vi "Accel math.vi"(4 "Numeric":i32, 8 "Base Accels 2":dbl[][](array[numeric]), 11 "Six Plane Accels 2":dbl[][](array[numeric])) -> (3 "Final Accel Values":dbl[][](array[numeric]))   [LabVIEW 2013]
uses:
  <vilib>/Analysis/NI_AALBase.lvlib
  <vilib>/Analysis/baseanly.llb/Real A x B.vi
  <vilib>/Analysis/baseanly.llb/Real Inverse Matrix.vi
panel:
  out "Final Accel Values 1":dbl[][](array[numeric])
  out "Numeric 4":dbl
  out "Numeric 2":dbl
  out "Numeric 3":dbl
  out "Final Accel Values 5":dbl[][](array[numeric])
  out "Final Accel Values 4":dbl[][](array[numeric])
  out "Final Accel Values 3":dbl[][](array[numeric])
  out "Final Accel Values 2":dbl[][](array[numeric])
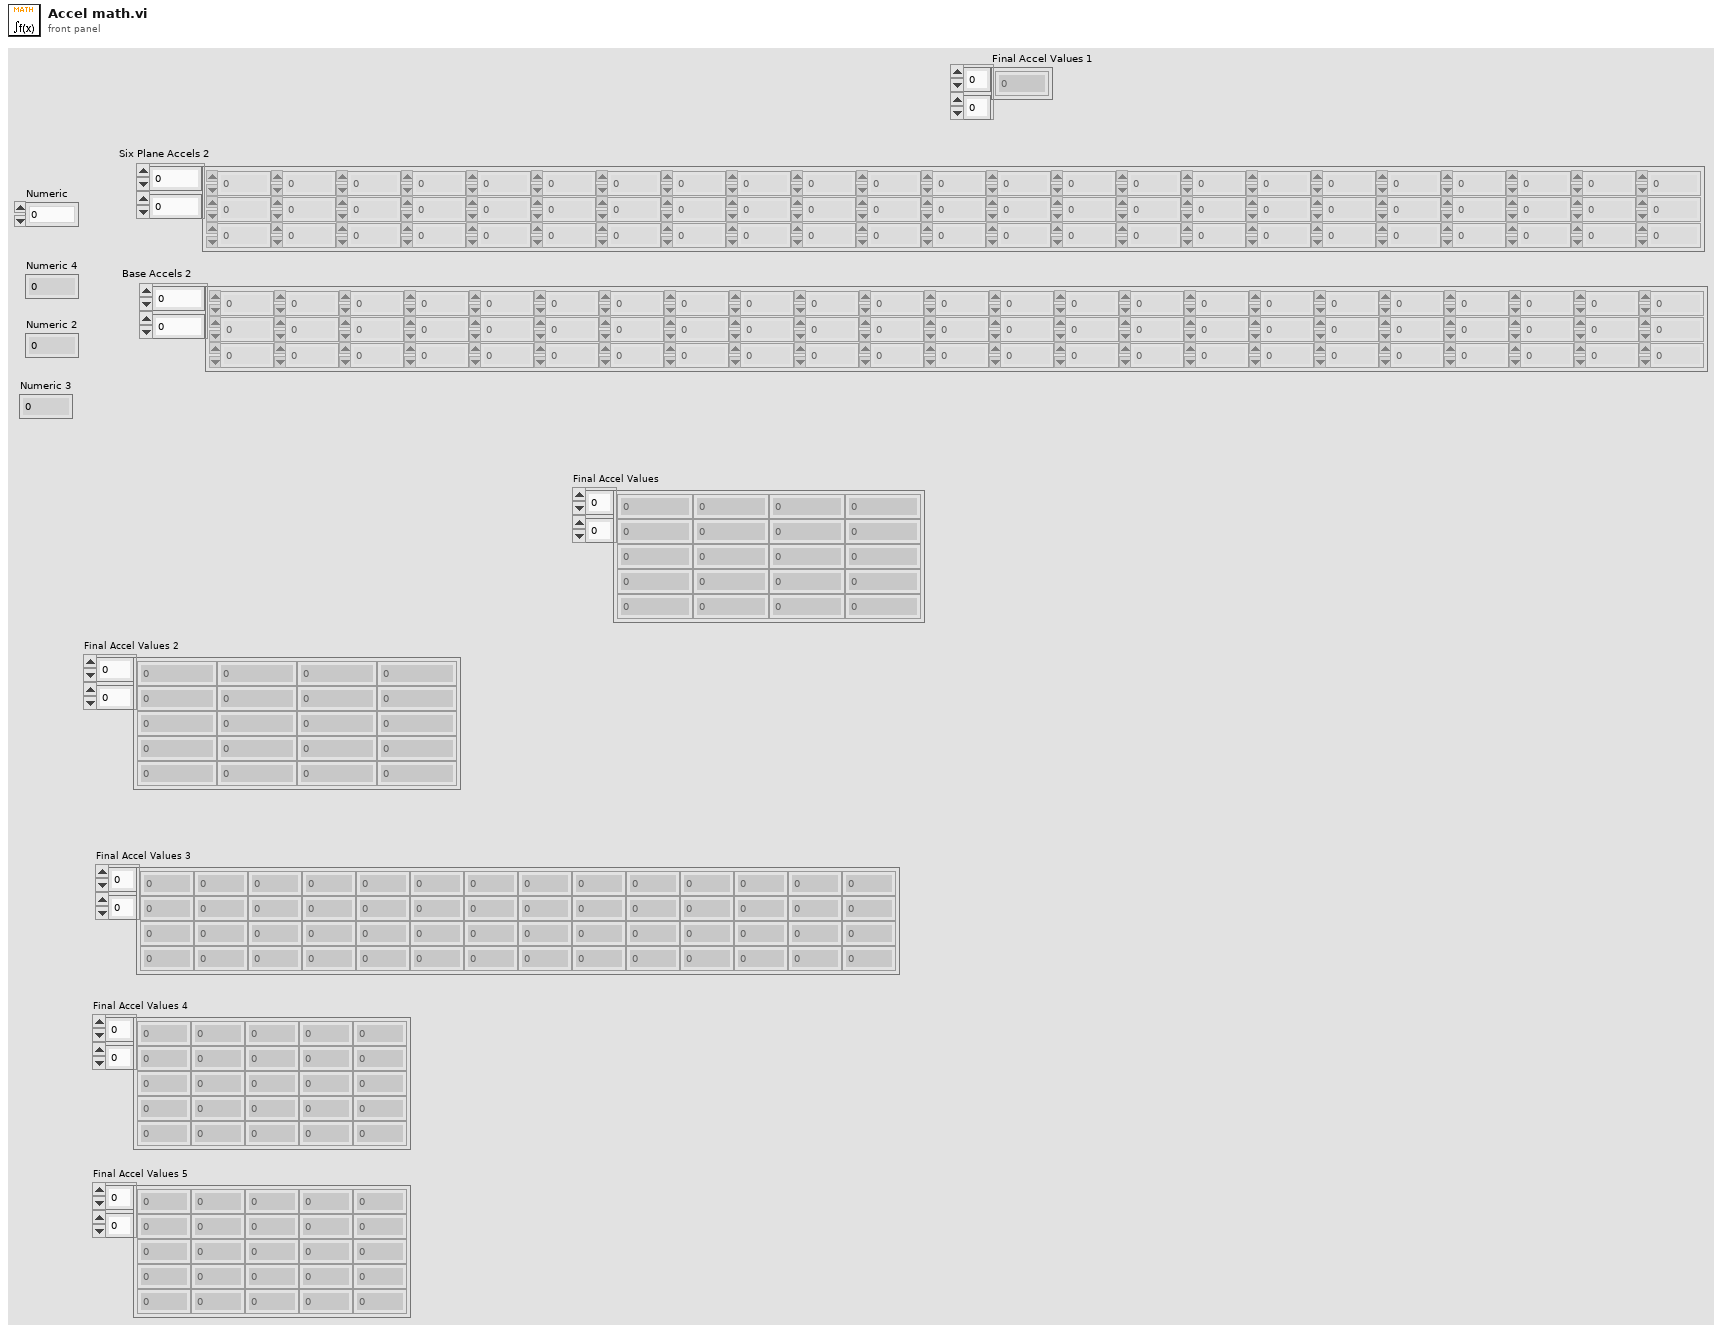
[diagram p1: front panel]
types:
  T1 = typedef "NI_Matrix.lvlib/RealMatrix.ctl" = dbl[][]
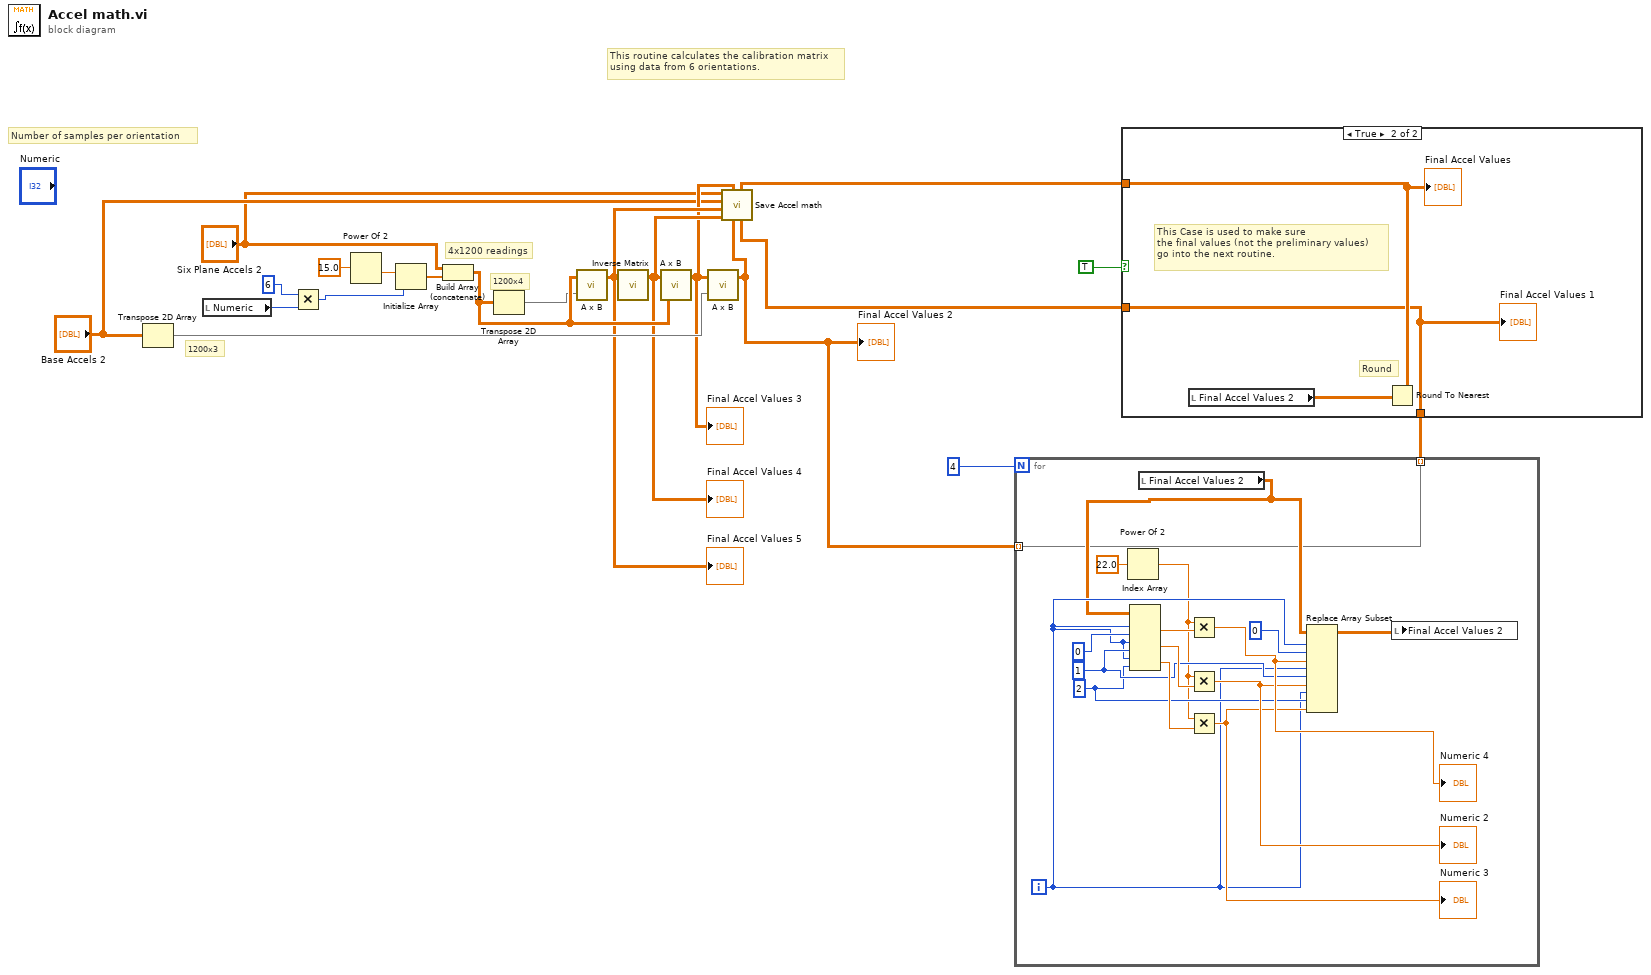
[diagram p0: block diagram]
diagram:
  # "This routine calculates the calibration matrix\nusing data from 6 orientations."
  # "Number of samples per orientation"
  # "1200x3"
  # "1200x4"
  # "4x1200 readings"
  n1 = Transpose 2D Array(2D array="Base Accels 2") -> (transposed array=w17:dbl[][])
  n2 = local read "Numeric"() -> (w2:i32)
  n3 = Multiply(x=6, y=w2) -> (x*y=w8:i32)
  n4 = Power Of 2(x=15.0) -> (2^x=w18:dbl)
  n5 = Initialize Array(w18, w8) -> (w20:dbl[])
  n6 = Build Array (concatenate)("Six Plane Accels 2", w20) -> (w16:dbl[][])
  n7 = Transpose 2D Array(2D array=w16) -> (transposed array=w15:dbl[][])
  n8 = call-poly <vilib>:"A x B.vi"("B"=w15, "A"=w16) -> ("A x B"=w14:T1)  [unwired: 1 out]
  "Final Accel Values 5" <- w14
  n9 = call-poly <vilib>:"Inverse Matrix.vi"("Input Matrix"=w14) -> ("Inverse Matrix"=w13:T1)  [unwired: 1 in, 1 out]
  "Final Accel Values 4" <- w13
  n10 = call-poly <vilib>:"A x B.vi"("B"=w16, "A"=w13) -> ("A x B"=w12:T1)  [unwired: 1 out]
  "Final Accel Values 3" <- w12
  n11 = call-poly <vilib>:"A x B.vi"("B"=w17, "A"=w12) -> ("A x B"=w6:T1)  [unwired: 1 out]
  "Final Accel Values 2" <- w6
  n12 = for {
    N: 4 -> [_]
    tunnel: w6 -> [w23] mode=indexing
    tunnel: [w23] -> w5 mode=indexing
    i -> [w26]
    w27 = 2
    w28 = 1
    n13 = Power Of 2(x=22.0) -> (2^x=w21:dbl)
    n14 = local read "Final Accel Values 2"() -> (w24:dbl[][])
    n15 = Index Array(array=w24, index (row) #1=w26, index (col) #1=0, index (row) #2=w26, index (col) #2=w28, index (row) #3=w26, index (col) #3=w27) -> (element #1=w35:dbl, element #2=w33:dbl, element #3=w32:dbl)
    n16 = Multiply(x=w21, y=w35) -> (x*y=w34:dbl)
    "Numeric 4" <- w34
    n17 = Multiply(x=w21, y=w33) -> (x*y=w31:dbl)
    "Numeric 2" <- w31
    n18 = Multiply(x=w21, y=w32) -> (x*y=w30:dbl)
    "Numeric 3" <- w30
    n19 = Replace Array Subset(array=w24, new element #1=w34, index (row) #1=w26, index (col) #1=0, new element #2=w31, index (row) #2=w26, index (col) #2=w28, new element #3=w30, index (row) #3=w26, index (col) #3=w27) -> (w25:dbl[][])
    n20 = local write "Final Accel Values 2"(w25) -> ()
  }
  n21 = case shown="True" TRUE {
    tunnel: w5 -> [w37 w38]
    tunnel: [w37 w39] -> w4
    tunnel: [w37 w38] -> w1
    frame False {
    }
    frame True {
      # "This Case is used to make sure\nthe final values (not the preliminary values) \ngo into the next routine."
      # "Round"
      n22 = local read "Final Accel Values 2"() -> (w40:dbl[][])
      n23 = Round To Nearest(number=w40) -> (nearest integer value=w39:dbl[][])
      "Final Accel Values" <- w39
      "Final Accel Values 1" <- w38
    }
  }
  n24 = call "Save Accel math.vi"("Final Accel Values"=w1, "Final Accel Values 1"=w4, "Final Accel Values 2"=w6, "Final Accel Values 3"=w12, "Final Accel Values 4"=w13, "Final Accel Values 5"=w14, "Base Accels"="Base Accels 2", "Six Plane Accels"="Six Plane Accels 2") -> ()  [unwired: 4 in]
